vi "setFreq.vi"(3 "error in":errorcluster, 5 "Frequenz in Hz":dbl=200.0 format="%.2f") -> (0 "error out":errorcluster)   [LabVIEW 2010]
panel:
  in  "mode (0)":i16
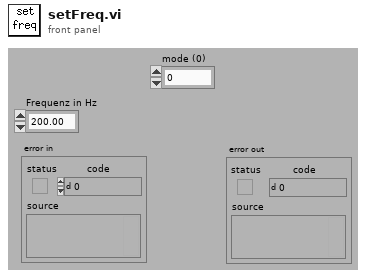
[diagram p1: front panel]
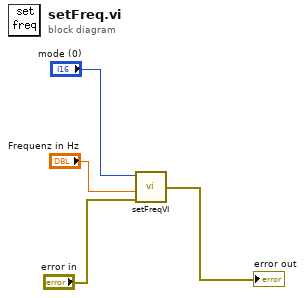
[diagram p0: block diagram]
diagram:
  n1 = call "setFreqVI.vi"("error in"="error in", "Frequenz in Hz"="Frequenz in Hz", "mode (0)"="mode (0)") -> ("error out"=→"error out":errorcluster)  [unwired: 1 in]
